vi "CSC_CalcCableLocFromCuff.vi"(8 "error in (no error)":errorcluster, 11 "C-Alex":refnum<class "CableSerialChain.lvclass">) -> (0 "error out":errorcluster, 3 "C-Alex Out":refnum<class "CableSerialChain.lvclass">)   [LabVIEW 2015, in "CableSerialChain.lvclass"]
uses:
  CableSerialChain.lvclass
  Cable.ctl
  Body/PointOnBody.ctl
  CableSerialChain.lvclass/CableSerialChain.ctl
  <vilib>/Analysis/BLAS.llb/dgemv - General Matrix-Vector Product (DBL).vi
  Body/Bodies.lvclass
  <vilib>/Analysis/NI_AALBLAS.lvlib
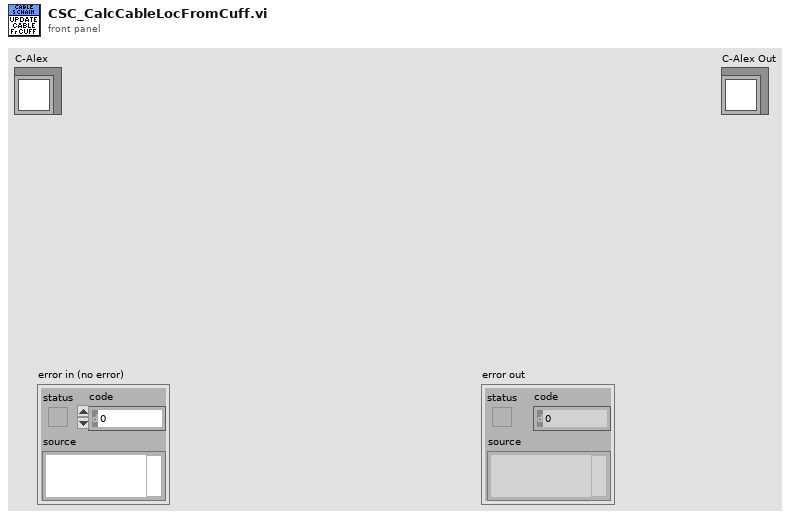
[diagram p1: front panel]
types:
  T1 = typedef "CableSerialChain.lvclass/Cable.ctl" = cluster{"RoutingPtsInLCS":T2[], "Cable ID":i32, "ActiveSegments":i32[][]}
  T2 = typedef "Bodies.lvclass/PointOnBody.ctl" = cluster{"Coord4":dbl[], "ID":i32}
  T3 = typedef "CableSerialChain.lvclass/Cuff.ctl" = cluster{"BodyID":i32, "CoM(CuffCS)":T2, "Mass(kg)":dbl, "CablePts(CuffCS)":T2[], "Cuff->Body":T4}
  T4 = typedef "NI_Matrix.lvlib/RealMatrix.ctl" = dbl[][]
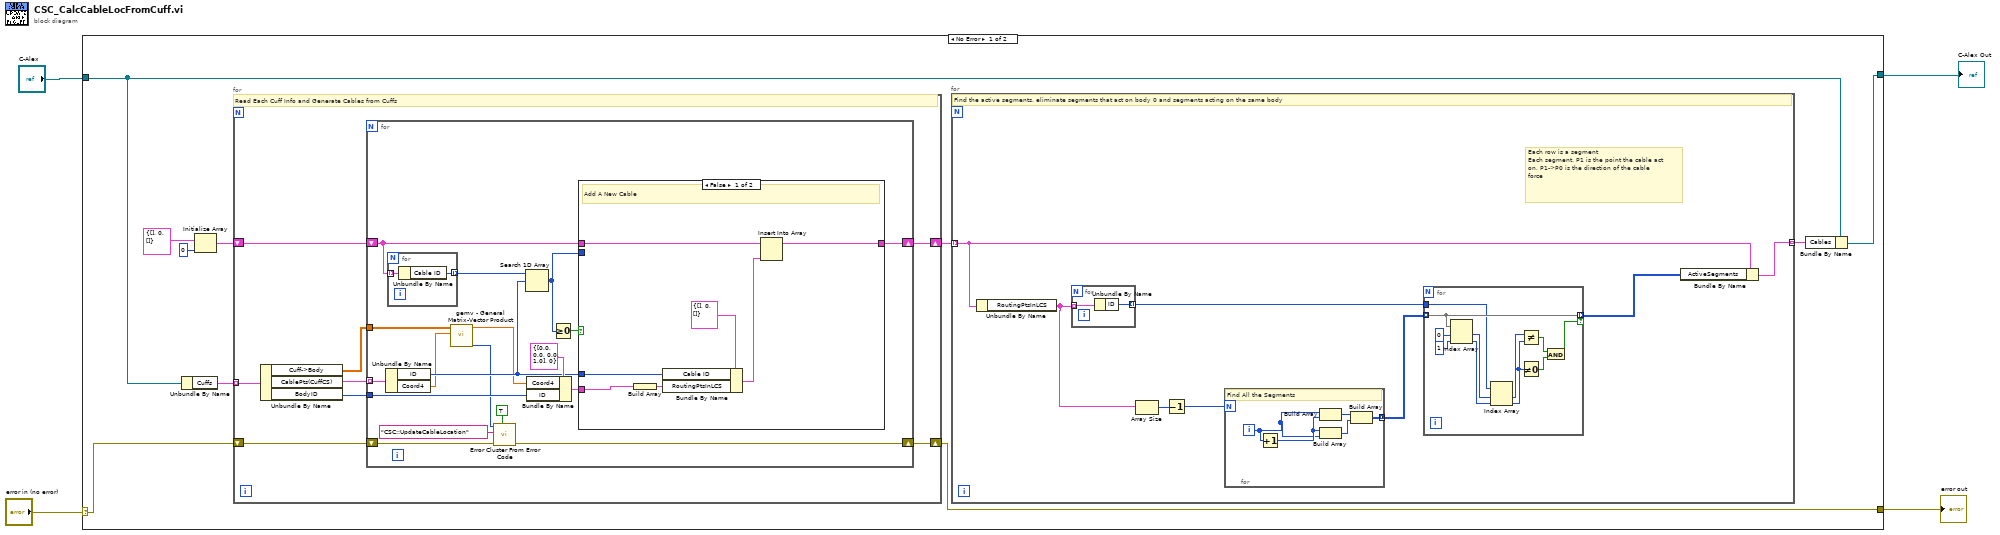
[diagram p0: block diagram]
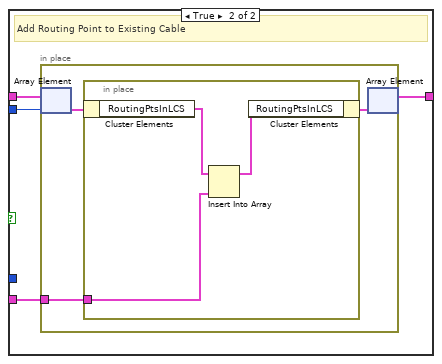
[diagram p2: hidden frame]
diagram:
  n1 = case shown="No Error" "error in (no error)" {
    selector: "error in (no error)" -> [w8 w87]
    tunnel: [w6 w87] -> w3
    tunnel: [w10 w86] -> w1
    tunnel: "C-Alex" -> [w13 w86]
    frame No Error {
      n2 = Unbundle By Name(w13) -> ("Cuffs"=w14:T3[])
      n3 = Initialize Array(T1 {"RoutingPtsInLCS"=[], "Cable ID"=0, "ActiveSegments"=[]} ("Cable"), 0 ("dimension size")) -> (w12:T1[])
      n4 = for {
        tunnel: w14 -> [w48] mode=indexing
        shift-right: [w44] -> w7
        shift-left: w12 -> [w45]
        shift-right: [w41] -> w6
        shift-left: w8 -> [w42]
        # "Read Each Cuff Info and Generate Cables from Cuffs"
        n5 = Unbundle By Name(w48) -> ("Cuff->Body"=w43:T4, "CablePts(CuffCS)"=w47:T2[], "BodyID"=w46:i32)
        n6 = for {
          tunnel: w47 -> [w66] mode=indexing
          tunnel: w46 -> [w64]
          shift-right: [w59] -> w44
          shift-left: w45 -> [w57]
          tunnel: w43 -> [w56]
          shift-right: [w51] -> w41
          shift-left: w42 -> [w52]
          n7 = Unbundle By Name(w66) -> ("ID"=w58:i32, "Coord4"=w55:dbl[])
          n8 = for {
            tunnel: w57 -> [w85] mode=indexing
            tunnel: [w84] -> w63 mode=indexing
            n9 = Unbundle By Name(w85) -> ("Cable ID"=w84:i32)
          }
          n10 = call-poly <vilib>:"gemv - General Matrix-Vector Product.vi"("x"=w55, "A"=w56) -> ("error"=w53:i32, "dgemv"=w54:dbl[])  [unwired: 8 in]
          n11 = call <vilib>:"Error Cluster From Error Code.vi"("show call chain? (False)"=TRUE, "error in (no error)"=w52, "error message (\"\")"="CSC::UpdateCableLocation" ("error message (\"\")"), "error code (0)"=w53) -> ("error out"=w51:errorcluster)  [unwired: 5 in]
          n12 = Search 1D Array(1D array=w63, element=w58) -> (index of element=w61:i32)  [unwired: 1 in]
          n13 = Bundle By Name(cluster=T2 {"Coord4"=[0.0, 0.0, 0.0, 1.0], "ID"=0} ("Point"), "Coord4"=w54, "ID"=w64) -> (w60:T2)
          n14 = Greater Or Equal To 0?(x=w61) -> (x >= 0?=w62:bool)
          n15 = case shown="False" w62 {
            tunnel: w61 -> [_ w76]
            tunnel: w57 -> [w73 w77]
            tunnel: w60 -> [w69 w74]
            tunnel: [w71 w75] -> w59
            tunnel: w58 -> [w72 _]
            frame False {
              # "Add A New Cable"
              n16 = Build Array(w69) -> (w67:T2[])
              n17 = Bundle By Name(cluster=T1 {"RoutingPtsInLCS"=[], "Cable ID"=0, "ActiveSegments"=[]} ("Cable"), "Cable ID"=w72, "RoutingPtsInLCS"=w67) -> (w70:T1)
              n18 = Insert Into Array(array=w73, new element=w70) -> (w71:T1[])  [unwired: 1 in]
            }
            frame True {
              # "Add Routing Point to Existing Cable"
              n19 = in-place {
                in-place-border: w74 -> [w79]
                n20 = in-place-array #1(w77, w76) -> (w80:T1)
                n21 = in-place {
                  in-place-border: w79 -> [w82]
                  n22 = in-place-cluster #2(w80) -> ("RoutingPtsInLCS"=w83:T2[])
                  n23 = Insert Into Array(array=w83, new element=w82) -> (w81:T2[])  [unwired: 1 in]
                  n24 = in-place-cluster #2("RoutingPtsInLCS"=w81) -> (w78:T1)
                }
                n25 = in-place-array #1(w78) -> (w75:T1[])  [unwired: 1 out]
              }
            }
          }
        }
      }
      n26 = for {
        tunnel: w7 -> [w22] mode=indexing
        tunnel: [w21] -> w5 mode=indexing
        # "Each row is a segment\nEach segment, P1 is the point the cable act on, P1->P0 is the direction of the cable force"
        # "Find the active segments, eliminate segments that act on body 0 and segments acting on the same body"
        n27 = Unbundle By Name(w22) -> ("RoutingPtsInLCS"=w18:T2[])
        n28 = for {
          tunnel: w18 -> [w40] mode=indexing
          tunnel: [w39] -> w15 mode=indexing
          n29 = Unbundle By Name(w40) -> ("ID"=w39:i32)
        }
        n30 = Array Size(array=w18) -> (size(s)=w19:i32)
        n31 = Decrement(x=w19) -> (x-1=w17:i32)
        n32 = for {
          N: w17 -> [_]
          tunnel: [w27] -> w16 mode=concatenating
          i -> [w23]
          # "Find All the Segments"
          n33 = Increment(x=w23) -> (x+1=w24:i32)
          n34 = Build Array(w23, w24) -> (w25:i32[])
          n35 = Build Array(w24, w23) -> (w26:i32[])
          n36 = Build Array(w25, w26) -> (w27:i32[][])
        }
        n37 = for {
          tunnel: w16 -> [w38] mode=indexing
          tunnel: [w38] -> w20 mode=indexing if=w33
          tunnel: w15 -> [w28]
          n38 = Index Array(array=w38, index #1=0 ("index"), index #2=1 ("index")) -> (element #1=w30:i32, element #2=w32:i32)
          n39 = Index Array(array=w28, index #1=w30, index #2=w32) -> (element #1=w29:i32, element #2=w31:i32)
          n40 = Not Equal?(x=w29, y=w31) -> (x != y?=w34:bool)
          n41 = Not Equal To 0?(x=w31) -> (x != 0?=w35:bool)
          n42 = And(x=w34, y=w35) -> (x .and. y?=w33:bool)
        }
        n43 = Bundle By Name(cluster=w22, "ActiveSegments"=w20) -> (w21:T1)
      }
      n44 = Bundle By Name(cluster=w13, "Cables"=w5) -> (w10:refnum<class "CableSerialChain.lvclass">)
    }
    frame Error {
    }
  }
  "error out" <- w3
  "C-Alex Out" <- w1
